vi "FT_CreateDevieInfoList.vi"() -> (0 "lpdwNumDevs":u32, 1 "FT_Status":u32)   [LabVIEW 2010]
uses:
  FTD2XX.dll
panel:
  # "Return the number of connected\nFTDI devices."
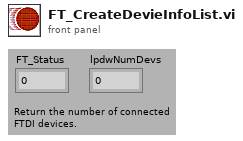
[diagram p1: front panel]
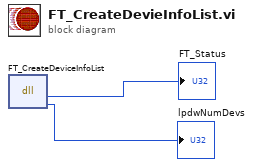
[diagram p0: block diagram]
diagram:
  n1 = dll-call lib="FTD2XX.dll" fn="FT_CreateDeviceInfoList"() -> ("FT_Status"=→"FT_Status":u32, "lpdwNumDevs"=→"lpdwNumDevs":u32)  [unwired: 4 in, 2 out]
